vi "testserver.vi"() -> ()   [LabVIEW 2016]
uses:
  dllwrapper/tls data user event.ctl
  dllwrapper/tls new socket user event.ctl
  dllwrapper/async tls.lvlib
  lvasynctls.dll
panel:
  out "errstring":string
  out "anyconn 2":u32 format="%.0x"
  out "anyconn":u64 format="%.0x"
  out "options":errorcluster
  out "data":string
  out "bad connection":u64
  out "request type 3":u8 format="%.0x"
  out "request ID 3":u32 format="%.0x"
  out "error code 3":i32 format="%.0x"
  out "request type 2":u8 format="%.0x"
  out "request ID 2":u32 format="%.0x"
  out "error code 2":i32 format="%.0x"
  out "error code":i32
  out "request ID":u32 format="%.0x"
  out "request type":u32 format="%.0x"
  out "error out 10":errorcluster
  out "error out 9":errorcluster
  out "error out 6":errorcluster
  out "error out 5":errorcluster
  out "error out 4":errorcluster
  out "error out 3":errorcluster
  out "error out 2":errorcluster
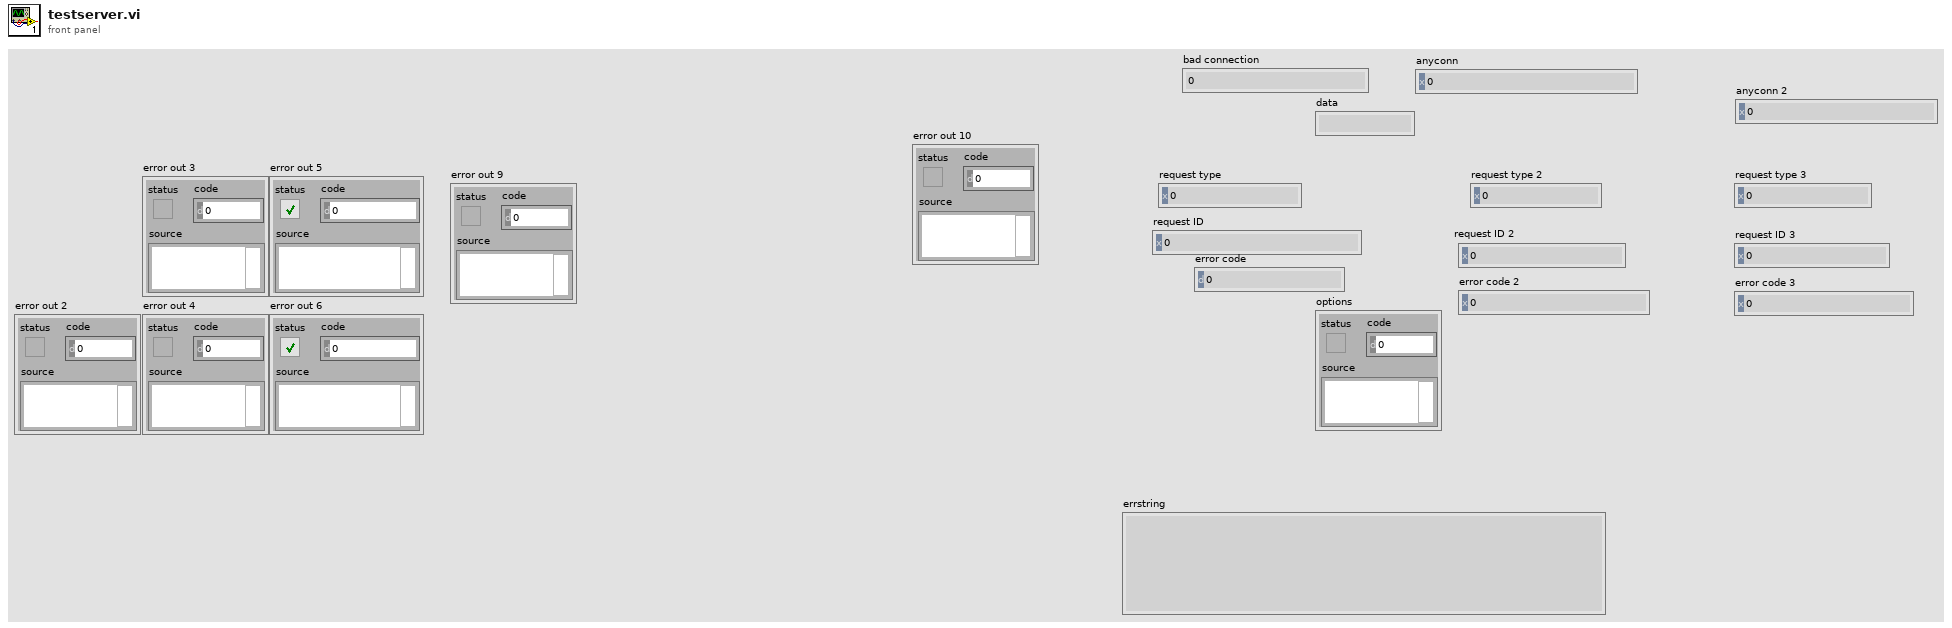
[diagram p1: front panel]
types:
  T1 = typedef "async tls.lvlib/tls new socket user event.ctl" = cluster{"request type":u32, "request ID":u32, "error code":i32, "errstring":string, "connection":u64}
  T2 = typedef "async tls.lvlib/tls data user event.ctl" = cluster{"request type":u8, "request ID":u32, "error code":i32, "data":string}
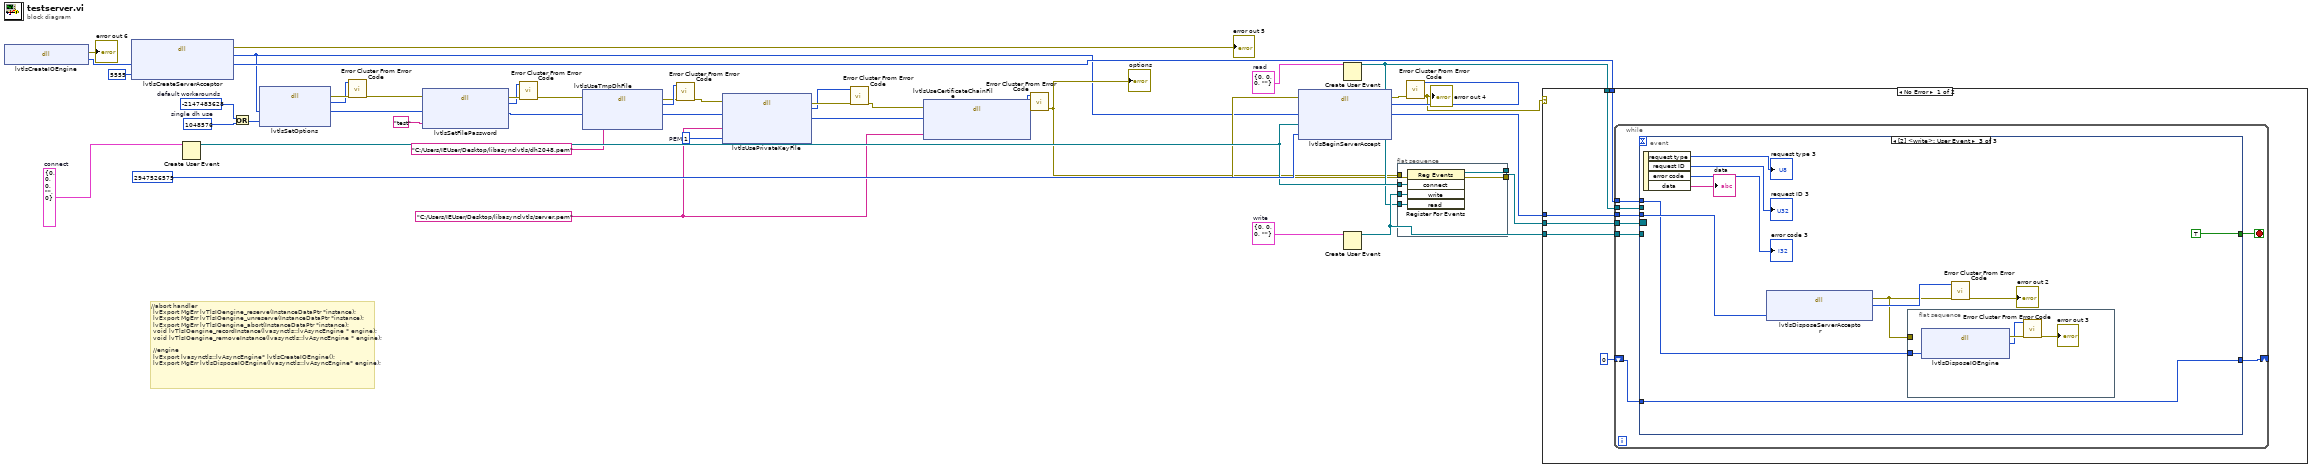
[diagram p0: block diagram]
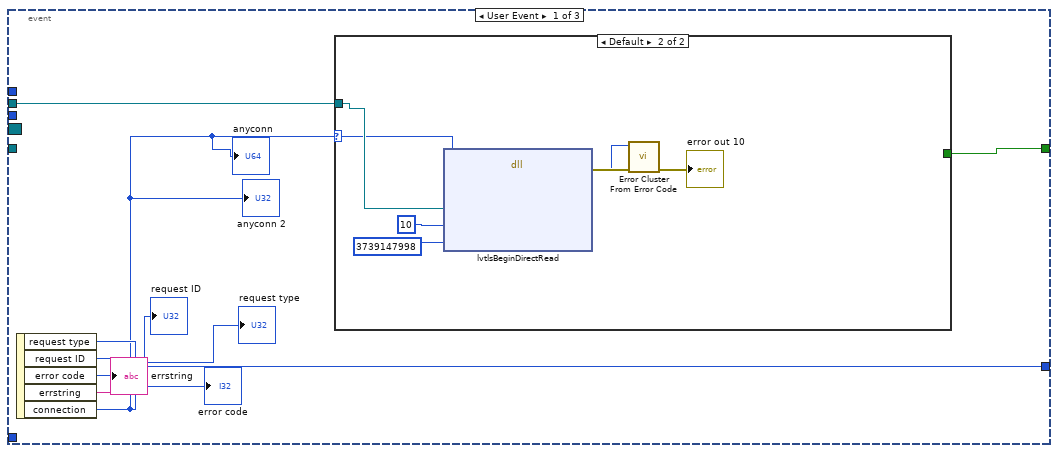
[diagram p2: hidden frame]
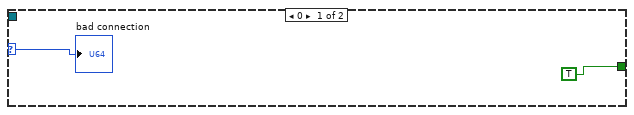
[diagram p3: hidden frame]
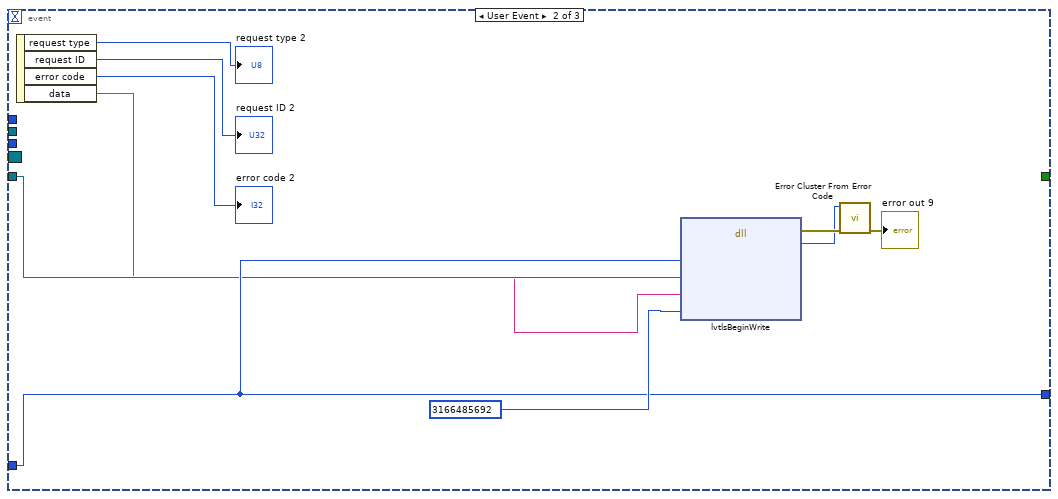
[diagram p4: hidden frame]
diagram:
  w11 = "C:/Users/IEUser/Desktop/libasynclvtls/server.pem" ("file")
  w13 = 1  # PEM
  w14 = -2147483628  # default workarounds
  w15 = 1048576  # single dh use
  w32 = T1 {"request type"=0, "request ID"=0, "error code"=0, "errstring"="", "connection"=0}  # connect
  w39 = T2 {"request type"=0, "request ID"=0, "error code"=0, "data"=""}  # read
  w38 = T2 {"request type"=0, "request ID"=0, "error code"=0, "data"=""}  # write
  # "//abort handler\n\tlvExport MgErr lvTlsIOengine_reserve(InstanceDataPtr *instance);\n\tlvExport MgErr lvTlsIOengine_unreserve(InstanceDataPtr *instance);\n\tlvExport MgErr lvTlsIOengine_abort(InstanceDataPtr *instance);\n\tvoid lvTlsIOengine_recordInstance(lvasynctls::lvAsyncEngine * engine);\n\tvoid lvTlsIOengine_removeInstance(lvasynctls::lvAsyncEngine * engine);\n\n\t//engine\n\tlvExport lvasynctls::lvAsyncEngine* lvtlsCreateIOEngine();\n\tlvExport MgErr lvtlsDisposeIOEngine(lvasynctls::lvAsyncEngine* engine);"
  n1 = dll-call lib="C:/Users/IEUser/Desktop/libasynclvtls/lvasynctls.dll" fn="lvtlsCreateIOEngine"() -> (error out=→"error out 6":errorcluster, "engine"=w45:u64)  [unwired: 3 in, 1 out]
  n2 = dll-call lib="C:/Users/IEUser/Desktop/libasynclvtls/lvasynctls.dll" fn="lvtlsCreateServerAcceptor"("engine"=w45, "port"=u16 5555) -> (error out=→"error out 5":errorcluster, "acceptor"=w2:u64, "engine"=w19:u64)  [unwired: 4 in, 1 out]
  n3 = Create User Event(user event datatype=w32) -> (user event=w35:refnum<user-event>)  [unwired: 1 in, 1 out]
  n4 = Or(x=w14, y=w15) -> (x .or. y?=w16:i32)
  n5 = dll-call lib="C:/Users/IEUser/Desktop/libasynclvtls/lvasynctls.dll" fn="lvtlsSetOptions"("connCreator"=w2, "options"=w16) -> (error out=w29:errorcluster, "err"=w28:i32, "connCreator"=w5:u64)  [unwired: 4 in, 1 out]
  n6 = call <vilib>:"Error Cluster From Error Code.vi"("error in (no error)"=w29, "error code (0)"=w28) -> ("error out"=w6:errorcluster)  [unwired: 7 in]
  n7 = dll-call lib="C:/Users/IEUser/Desktop/libasynclvtls/lvasynctls.dll" fn="lvtlsSetFilePassword"(error in=w6, "connCreator"=w5, "password"="test" ("file")) -> (error out=w9:errorcluster, "err"=w8:i32, "connCreator"=w4:u64)  [unwired: 3 in, 1 out]
  n8 = call <vilib>:"Error Cluster From Error Code.vi"("error in (no error)"=w9, "error code (0)"=w8) -> ("error out"=w7:errorcluster)  [unwired: 7 in]
  n9 = dll-call lib="C:/Users/IEUser/Desktop/libasynclvtls/lvasynctls.dll" fn="lvtlsUseTmpDhFile"(error in=w7, "connCreator"=w4, "file"="C:/Users/IEUser/Desktop/libasynclvtls/dh2048.pem") -> (error out=w26:errorcluster, "err"=w27:i32, "connCreator"=w18:u64)  [unwired: 3 in, 1 out]
  n10 = call <vilib>:"Error Cluster From Error Code.vi"("error in (no error)"=w26, "error code (0)"=w27) -> ("error out"=w20:errorcluster)  [unwired: 7 in]
  n11 = dll-call lib="C:/Users/IEUser/Desktop/libasynclvtls/lvasynctls.dll" fn="lvtlsUsePrivateKeyFile"(error in=w20, "connCreator"=w18, "file"=w11, "format"=w13) -> (error out=w25:errorcluster, "err"=w24:i32, "connCreator"=w17:u64)  [unwired: 4 in, 1 out]
  n12 = call <vilib>:"Error Cluster From Error Code.vi"("error in (no error)"=w25, "error code (0)"=w24) -> ("error out"=w21:errorcluster)  [unwired: 7 in]
  n13 = dll-call lib="C:/Users/IEUser/Desktop/libasynclvtls/lvasynctls.dll" fn="lvtlsUseCertificateChainFile"(error in=w21, "connCreator"=w17, "file"=w11) -> (error out=w22:errorcluster, "err"=w23:i32)  [unwired: 4 in, 1 out]
  n14 = call <vilib>:"Error Cluster From Error Code.vi"("error in (no error)"=w22, "error code (0)"=w23) -> ("error out"=w12:errorcluster)  [unwired: 7 in]
  "options" <- w12
  n15 = dll-call lib="C:/Users/IEUser/Desktop/libasynclvtls/lvasynctls.dll" fn="lvtlsBeginServerAccept"(error in=w31, "acceptor"=w2, "event"=w35, "id"=u32 2947526575 ("err")) -> (error out=w43:errorcluster, "err"=w37:i32, "acceptor"=w36:u64)  [unwired: 4 in, 1 out]
  n16 = Create User Event(user event datatype=w39) -> (user event=w33:refnum<user-event>)  [unwired: 1 in, 1 out]
  n17 = Create User Event(user event datatype=w38) -> (user event=w34:refnum<user-event>)  [unwired: 1 in, 1 out]
  n18 = flat-sequence {
    tunnel: [w50] -> w40
    tunnel: w35 -> [w49]
    tunnel: w34 -> [w48]
    tunnel: w33 -> [w47]
    tunnel: [w46] -> w31
    tunnel: w12 -> [_]
    frame #0 {
      n19 = register-events(w49, w48, w47) -> (reference out=w50:refnum<event-registration>, error out=w46:errorcluster)  [unwired: 2 in]
    }
  }
  n20 = call <vilib>:"Error Cluster From Error Code.vi"("error in (no error)"=w43, "error code (0)"=w37) -> ("error out"=w1:errorcluster)  [unwired: 7 in]
  "error out 4" <- w1
  n21 = case shown="No Error" w1 {
    tunnel: w40 -> [w56 _]
    tunnel: w36 -> [w55 _]
    tunnel: w34 -> [w54 _]
    tunnel: w33 -> [w53 _]
    tunnel: w19 -> [w51 _]
    frame No Error {
      n22 = while {
        tunnel: w56 -> [w64]
        tunnel: w54 -> [w62]
        tunnel: w55 -> [w61]
        tunnel: w53 -> [w60]
        tunnel: w51 -> [w59]
        shift-right: [w58] -> _
        shift-left: u32 0 -> [w57]
        stop <- w63 stop-if-true
        n23 = event shown="[2] <write>: User Event" {
          selector: w64 -> [_ _ _]
          dyn-events: _ -> [_ _ _]
          timeout: _ -> [_ _ _]
          tunnel: [w68 _ TRUE] -> w63
          tunnel: w62 -> [_ w82 _]
          tunnel: w61 -> [_ _ w95]
          tunnel: w60 -> [w67 _ _]
          tunnel: w59 -> [_ _ w94]
          tunnel: [w66 w83 w92] -> w58
          tunnel: w57 -> [_ w83 w92]
          event User Event {
            n24 = event-data() -> ("request type"=→"request type":u32, "request ID"=→"request ID":u32, "error code"=→"error code":i32, "errstring"=→"errstring":string, "connection"=w66:u64)  [unwired: 1 in]
            "anyconn" <- w66
            "anyconn 2" <- w66
            n25 = case shown="Default" w66 {
              selector: w66 -> [w72 w74]
              tunnel: [TRUE _] -> w68
              tunnel: w67 -> [_ w75]
              frame 0 {
                "bad connection" <- w72
              }
              frame Default {
                n26 = dll-call lib="C:/Users/IEUser/Desktop/libasynclvtls/lvasynctls.dll" fn="lvtlsBeginDirectRead"("socket"=w74, "event"=w75, "bytes to read"=10, "id"=u32 3739147998 ("err")) -> (error out=w79:errorcluster, "err"=w77:i32)  [unwired: 7 in, 1 out]
                n27 = call <vilib>:"Error Cluster From Error Code.vi"("error in (no error)"=w79, "error code (0)"=w77) -> ("error out"=→"error out 10":errorcluster)  [unwired: 7 in]
              }
            }
          }
          event User Event {
            n28 = event-data() -> ("request type"=→"request type 2":u8, "request ID"=→"request ID 2":u32, "error code"=→"error code 2":i32, "data"=w81:string)  [unwired: 1 in]
            n29 = dll-call lib="C:/Users/IEUser/Desktop/libasynclvtls/lvasynctls.dll" fn="lvtlsBeginWrite"("socket"=w83, "event"=w82, "data"=w81, "requestID"=u32 3166485692 ("err")) -> (error out=w87:errorcluster, "err"=w85:i32)  [unwired: 7 in, 1 out]
            n30 = call <vilib>:"Error Cluster From Error Code.vi"("error in (no error)"=w87, "error code (0)"=w85) -> ("error out"=→"error out 9":errorcluster)  [unwired: 7 in]
          }
          event User Event {
            n31 = event-data() -> ("request type"=→"request type 3":u8, "request ID"=→"request ID 3":u32, "error code"=→"error code 3":i32, "data"=→"data":string)  [unwired: 1 in]
            n32 = dll-call lib="C:/Users/IEUser/Desktop/libasynclvtls/lvasynctls.dll" fn="lvtlsDisposeServerAcceptor"("acceptor"=w95) -> (error out=w93:errorcluster, "err"=w97:i32)  [unwired: 4 in, 1 out]
            n33 = flat-sequence {
              tunnel: w94 -> [w102]
              tunnel: w93 -> [_]
              frame #0 {
                n34 = dll-call lib="C:/Users/IEUser/Desktop/libasynclvtls/lvasynctls.dll" fn="lvtlsDisposeIOEngine"("engine"=w102) -> (error out=w105:errorcluster, "err"=w104:i32)  [unwired: 4 in, 1 out]
                n35 = call <vilib>:"Error Cluster From Error Code.vi"("error in (no error)"=w105, "error code (0)"=w104) -> ("error out"=→"error out 3":errorcluster)  [unwired: 7 in]
              }
            }
            n36 = call <vilib>:"Error Cluster From Error Code.vi"("error in (no error)"=w93, "error code (0)"=w97) -> ("error out"=→"error out 2":errorcluster)  [unwired: 7 in]
          }
        }
      }
    }
    frame Error {
    }
  }
